vi "MB_C843.21_init (Magnet Motors).vi"(11 "System no.":i32=1) -> (0 "error out":errorcluster, 2 "C843\nConn. \nAxis":string[](array[string]), 3 "Position":dbl[](array[numeric]) format="%.6f")   [LabVIEW 2011]
panel:
  in  "Board number":i32=1
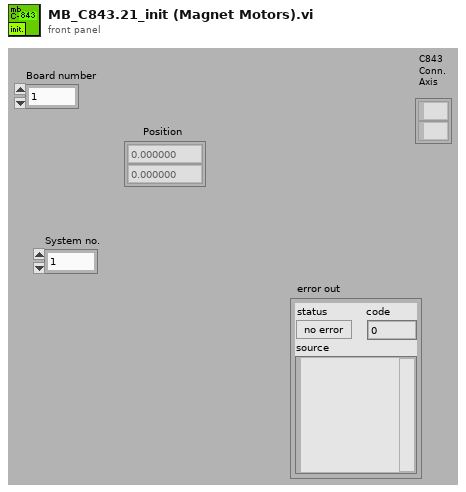
[diagram p1: front panel]
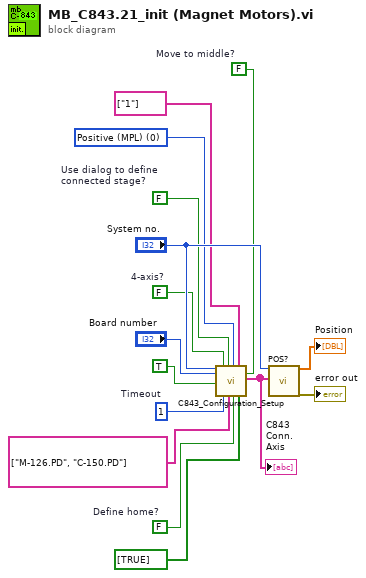
[diagram p0: block diagram]
diagram:
  w3 = FALSE  # Define home?
  w4 = u32 1  # Timeout
  w6 = FALSE  # Move to middle?
  w7 = u16 0 items=["Positive (MPL)", "Negative (MNL)"] ("Limit switch selection")
  w8 = FALSE  # 4-axis?
  w9 = FALSE  # Use dialog to define connected stage?
  n1 = call "C843_Configuration_Setup.vi"("System no."="System no.", "C-843 Board No."="Board number", "All axes?"=TRUE, "C-843 version"=w8, "Timeout"=w4, "Use dialog to define\nconnected stages?"=w9, "Stage names input"=string[] ["M-126.PD", "C-150.PD"] ("Stage name input"), "Limit switch selection"=w7, "Define home?"=w3, "RON Affected axes"=string[] ["1"], "Reference mode"=bool[] [TRUE], "Move to middle?"=w6) -> ("Conn. \nAxes"=w1:string[])  [unwired: 3 in, 4 out]
  "C843\nConn. \nAxis" <- w1
  n2 = call "POS?.vi"("System no."="System no.", "Axes to query"=w1) -> ("Position"=→"Position":dbl[], "error out"=→"error out":errorcluster)  [unwired: 3 in, 13 out]
